vi "RVHR - Set Image Size.vi"(8 "error in (no error)":errorcluster, 10 "Rectangle":T1, 11 "Image_L":refnum<vi>) -> (0 "error out":errorcluster)   [LabVIEW 2024]
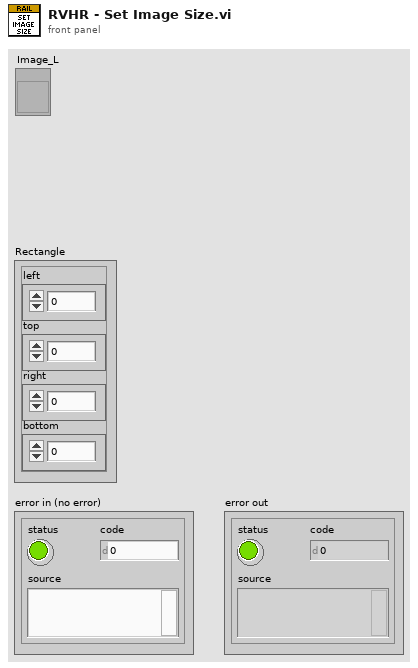
[diagram p1: front panel]
types:
  T1 = cluster{"left":i16, "top":i16, "right":i16, "bottom":i16}
  T2 = typedef "LVBoundsTypeDef.ctl" = cluster{"Width":u32, "Height":u32}
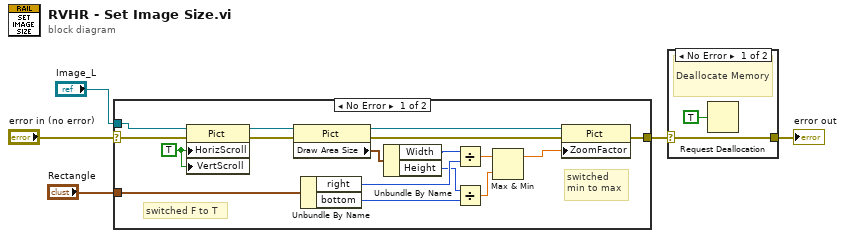
[diagram p0: block diagram]
diagram:
  n1 = case shown="No Error" "error in (no error)" {
    selector: "error in (no error)" -> [w9 w23]
    tunnel: "Image_L" -> [w11 _]
    tunnel: [w12 w23] -> w2
    tunnel: "Rectangle" -> [w22 _]
    frame No Error {
      w7 = TRUE ("Horizontal Scrollbar Visible")
      # "switched F to T"
      # "switched\nmin to max"
      n2 = property on="Property Node" class="Pict"(reference=w11, error in=w9, "HorizScroll"=w7, "VertScroll"=w7) -> (reference out=w10:refnum<vi>, error out=w8:errorcluster)
      n3 = property on="Property Node" class="Pict"(reference=w10, error in=w8) -> (reference out=w14:refnum<vi>, error out=w15:errorcluster, "Draw Area Size"=w13:T2)
      n4 = Unbundle By Name(w22) -> ("right"=w20:i16, "bottom"=w21:i16)
      n5 = Unbundle By Name(w13) -> ("Width"=w16:u32, "Height"=w17:u32)
      n6 = Divide(x=w16, y=w20) -> (x/y=w18:dbl)
      n7 = Divide(x=w17, y=w21) -> (x/y=w19:dbl)
      n8 = Max & Min(x=w18, y=w19) -> (max(x,y)=w6:dbl)  [unwired: 1 out]
      n9 = property on="Property Node" class="Pict"(reference=w14, error in=w15, "ZoomFactor"=w6) -> (error out=w12:errorcluster)  [unwired: 1 out]
    }
    frame Error {
    }
  }
  n10 = case shown="No Error" w2 {
    selector: w2 -> [w24 w26]
    tunnel: [w24 w26] -> w1
    frame No Error {
      # "Deallocate Memory"
      n11 = Request Deallocation(TRUE ("flag")) -> ()
    }
    frame Error {
    }
  }
  "error out" <- w1
